vi "Decode IDN query response.vi"(8 "error in (no error)":errorcluster, 11 "*IDN? result":string) -> (0 "error out":errorcluster, 1 "LECROY found?":bool, 3 "Series ID":u32, 5 "Instrument Information":T1)   [LabVIEW 2020, in "LeCroy Wave Series.lvlib"]
doc: "Decodes the response to the *IDN? query. Outputs an identifier for each class of LeCroy Oscilloscopes and a boolean = TRUE if the scope is found to be a LECROY by virtue of having the substring \"LECROY\" within the *IDN? response."
uses:
  LeCroy Wave Series.lvlib
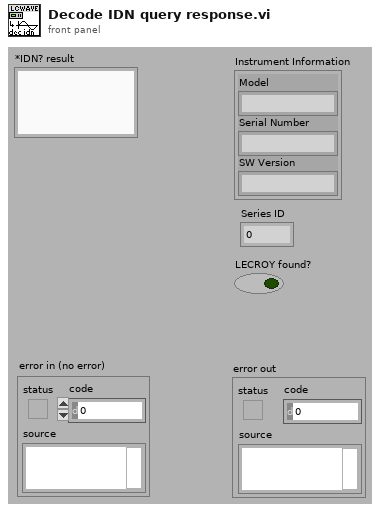
[diagram p1: front panel]
types:
  T1 = cluster{"Model":string, "Serial Number":string, "SW Version":string}
  T2 = cluster{"Status":bool, "Code":i32, "Source (VI Name)":string}
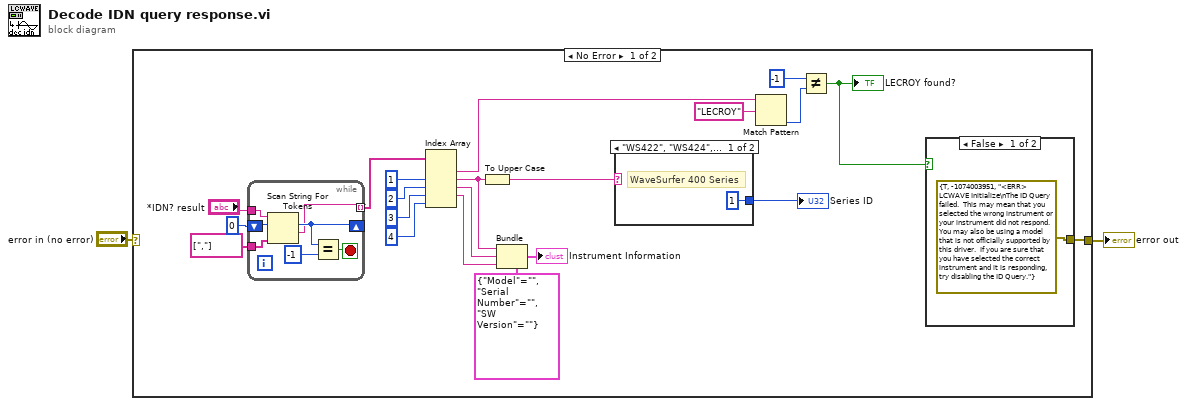
[diagram p0: block diagram]
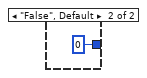
[diagram p3: hidden frame]
diagram:
  n1 = case shown="No Error" "error in (no error)" {
    selector: "error in (no error)" -> [_ w34]
    tunnel: [w4 w34] -> w1
    frame No Error {
      n2 = while {
        shift-right: [w29] -> _
        shift-left: 0 ("offset past token") -> [w31]
        tunnel: [w27] -> w17 mode=indexing
        tunnel: "*IDN? result" -> [w26]
        tunnel: string[] [","] ("delimiters (\\s,\\t,\\r,\\n)") -> [w25]
        stop <- w30 stop-if-true
        n3 = Scan String For Tokens(6:w25, 8:w31, 9:w26) -> (1:w27:string, 2:w29:i32)  [unwired: 3 in, 2 out]
        n4 = Equal?(x=w29, y=-1) -> (x = y?=w30:bool)
      }
      n5 = Index Array(array=w17, index #2=1 ("index"), index #3=2 ("index"), index #4=3 ("index"), index #5=4 ("index")) -> (element #1=w16:string, element #2=w10:string, element #3=w9:string, element #4=w8:string)  [unwired: 1 in, 1 out]
      n6 = To Upper Case(1:w10) -> (0:w6:string)
      n7 = Bundle(cluster=T1 {"Model"="", "Serial Number"="", "SW Version"=""} ("Instrument Information"), "Model"=w10, "Serial Number"=w9, "SW Version"=w8) -> (→"Instrument Information":T1)
      n8 = case shown="\"WS422\", \"WS424\", \"WS432\", \"WS434\", \"WS452'\", \"WS454\"" w6 {
        tunnel: [1 0] -> w5
        frame "WS422", "WS424", "WS432", "WS434", "WS452'", "WS454" {
          # "WaveSurfer 400 Series"
        }
        frame "False", Default {
        }
      }
      "Series ID" <- w5
      n9 = Match Pattern(string=w16, regular expression="LECROY") -> (offset past match=w22:i32)  [unwired: 1 in, 3 out]
      n10 = Not Equal?(x=-1, y=w22) -> (x != y?=w3:bool)
      "LECROY found?" <- w3
      n11 = case shown="False" w3 {
        tunnel: [T2 {"Status"=TRUE, "Code"=-1074003951, "Source (VI Name)"="<ERR> LCWAVE Initialize\nThe ID Query failed.  This may mean that you selected the wrong instrument or your instrument did not respond.  You may also be using a model that is not officially supported by this driver.  If you are sure that you have selected the correct instrument and it is responding, try disabling the ID Query."} _] -> w4
        frame False {
        }
        frame True {
        }
      }
    }
    frame Error {
    }
  }
  "error out" <- w1
